vi "ChangeUI.vi"(8 "error in (no error)":errorcluster caption="错误输入（无错误）", 10 "TreeTag":string, 11 "SubPnl*":refnum<vi>) -> (0 "error out":errorcluster caption="错误输出")   [LabVIEW 2016]
uses:
  FGV_ThreadsManager.ctl
  Modules/DAQ-Display/PanelSplitToolkit/QueueManager.llb/Insert.vi
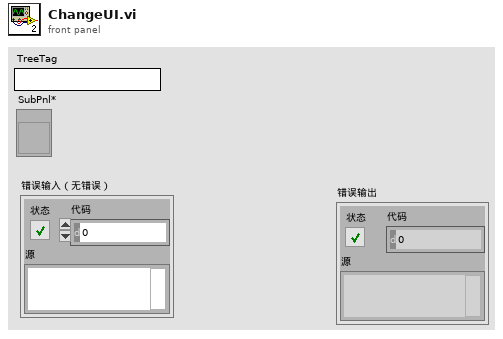
[diagram p1: front panel]
types:
  T1 = typedef "FGV_ThreadsManager.ctl" = enum16{"Load Threads", "GetVI*", "Other"}
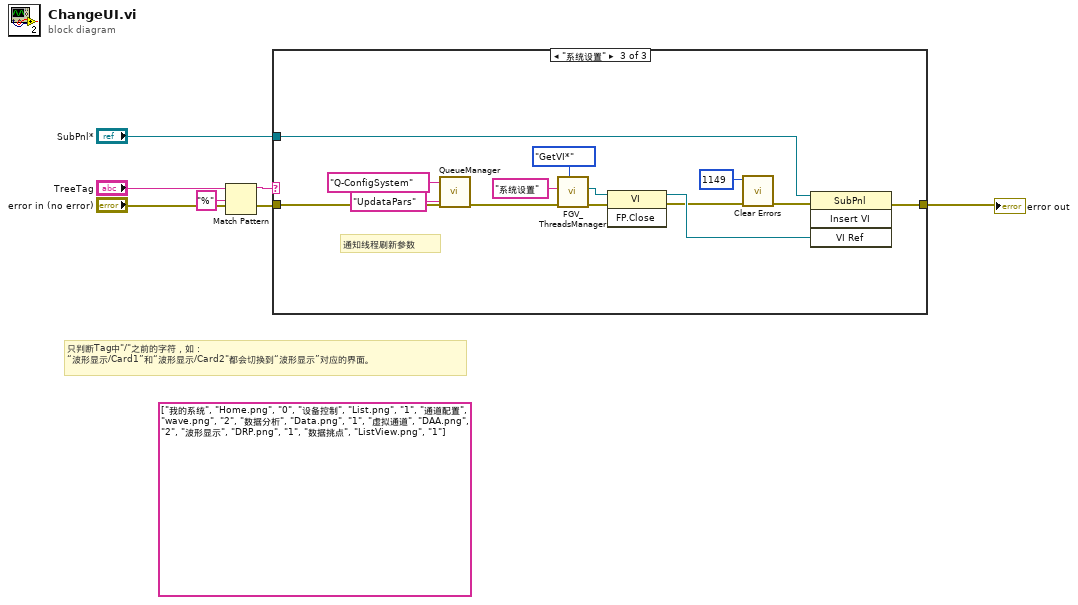
[diagram p0: block diagram]
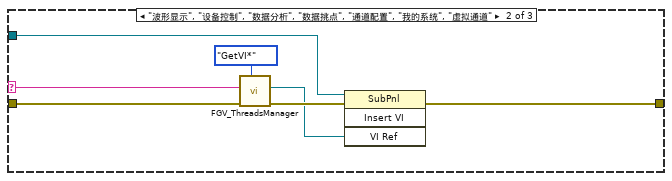
[diagram p3: hidden frame]
diagram:
  (unwired) string[][] [["我的系统", "Home.png", "0"], ["设备控制", "List.png", "1"], ["通道配置", "wave.png", "2"], ["数据分析", "Data.png", "1"], ["虚拟通道", "DAA.png", "2"], ["波形显示", "DRP.png", "1"], ["数据挑点", "ListView.png", "1"]]
  # "只判断Tag中\"/\"之前的字符，如：\n“波形显示/Card1”和“波形显示/Card2\"都会切换到“波形显示”对应的界面。"
  n1 = Match Pattern(string="TreeTag", regular expression="%" ("正则表达式")) -> (before substring=w1:string)  [unwired: 1 in, 3 out]
  n2 = case shown="\"系统设置\"" w1 {
    selector: w1 -> [_ w14 _]
    tunnel: "SubPnl*" -> [_ w12 w27]
    tunnel: "error in (no error)" -> [w7 w9 w24]
    tunnel: [w7 w8 w26] -> w4
    frame "假", Default {
    }
    frame "波形显示", "设备控制", "数据分析", "数据挑点", "通道配置", "我的系统", "虚拟通道" {
      n3 = call "FGV_ThreadsManager.vi"("Action"=FGV_ThreadsManager."GetVI*", "error in"=w9, "Tag"=w14) -> ("error out"=w11:errorcluster, "Vi*"=w10:refnum<vi>)  [unwired: 7 in]
      n4 = invoke on="调用节点" class="SubPnl" method="Insert VI"(reference=w12, error in=w11, "VI Ref"=w10) -> (error out=w8:errorcluster)  [unwired: 1 in, 3 out]
    }
    frame "系统设置" {
      # "通知线程刷新参数"
      n5 = call-poly "QueueManager.vi"("error in"=w24, "Event"="UpdataPars", "QueueName"="Q-ConfigSystem") -> ("error out"=w23:errorcluster)  [unwired: 7 in, 1 out]
      n6 = call "FGV_ThreadsManager.vi"("Action"=FGV_ThreadsManager."GetVI*", "error in"=w23, "Tag"="系统设置") -> ("error out"=w18:errorcluster, "Vi*"=w20:refnum<vi>)  [unwired: 7 in]
      n7 = invoke class="VI" method="FP.Close"(reference=w20, error in=w18) -> (reference out=w19:refnum<vi>, error out=w16:errorcluster)  [unwired: 1 in, 1 out]
      n8 = call <vilib>:"Clear Errors.vi"("error in (no error)"=w16, "specific error code to clear (0: all)"=1149) -> ("error out"=w15:errorcluster)  [unwired: 4 in, 1 out]
      n9 = invoke on="调用节点" class="SubPnl" method="Insert VI"(reference=w27, error in=w15, "VI Ref"=w19) -> (error out=w26:errorcluster)  [unwired: 1 in, 3 out]
    }
  }
  "error out" <- w4
